vi "Calculate H Score.vi"(7 "End":cluster{"Row":i32, "Col":i32}, 11 "Position":cluster{"Row":i32, "Col":i32}) -> (3 "hScore":i32)   [LabVIEW 2022 SP3, in "AoC22.lvlib"]
uses:
  AoC22.lvlib
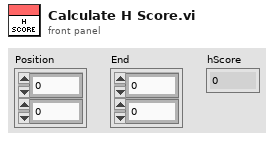
[diagram p1: front panel]
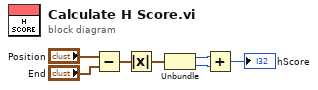
[diagram p0: block diagram]
diagram:
  n1 = Subtract(x="Position", y="End") -> (x-y=w5:cluster{"Row":i32, "Col":i32})
  n2 = Absolute Value(x=w5) -> (abs(x)=w4:cluster{"Row":i32, "Col":i32})
  n3 = Unbundle(w4) -> ("Row"=w3:i32, "Col"=w2:i32)
  n4 = Add(x=w3, y=w2) -> (x+y=→"hScore":i32)
